vi "CLD 1_Elapsed_Time_Express_ZLK_Solution.vi"(6 "Stop VI":bool, 8 "error in":errorcluster, 9 "Auto Reset":bool=TRUE, 10 "Reset Button":bool, 11 "Time Target (s)":dbl=2.0) -> (0 "error out":errorcluster, 2 "Time has Elapsed":bool, 3 "Elapsed Time":string="0  00:00:00")   [LabVIEW 2023]
doc: "LabVIEW CLD 1 Exercise"
uses:
  b5ba48de-fc09-4468-998c-c920f8fd6674.vi
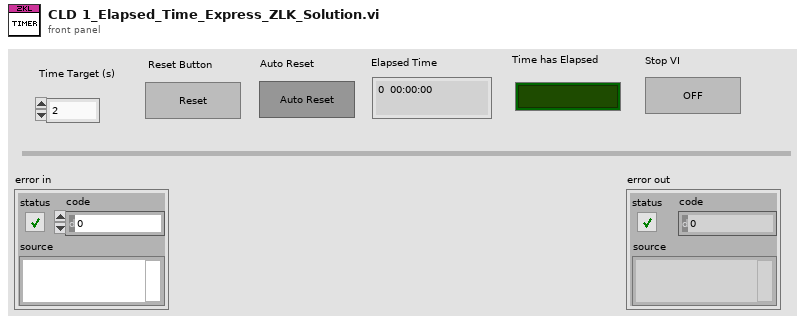
[diagram p1: front panel]
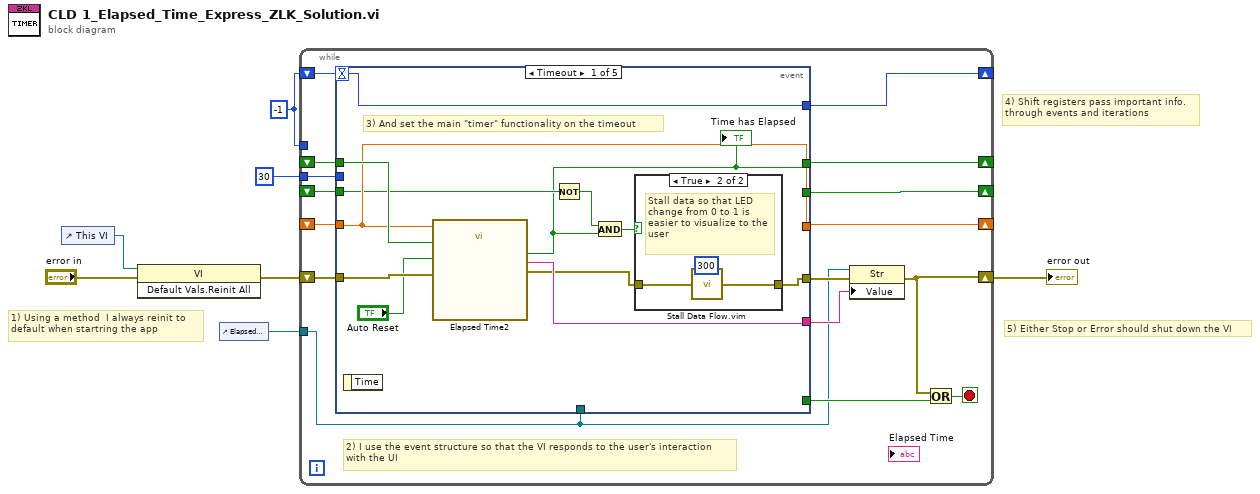
[diagram p0: block diagram]
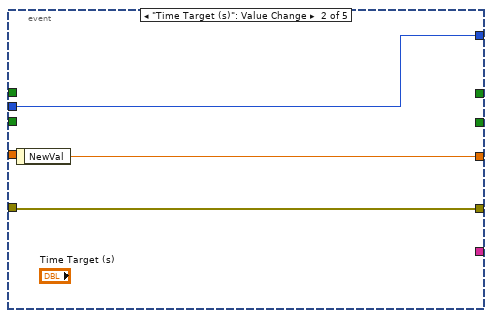
[diagram p3: hidden frame]
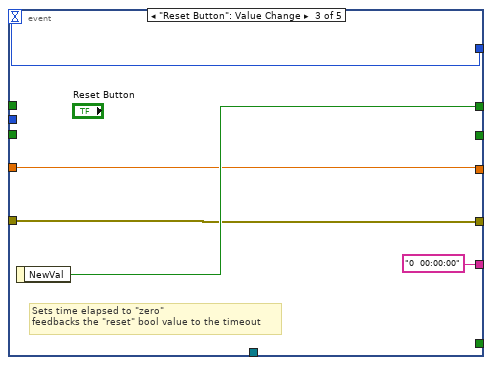
[diagram p4: hidden frame]
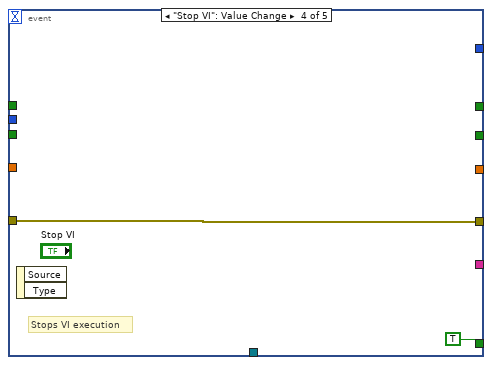
[diagram p5: hidden frame]
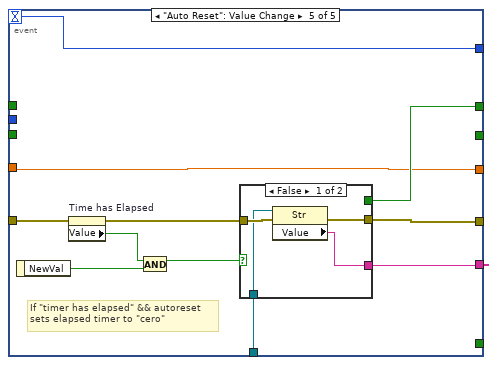
[diagram p6: hidden frame]
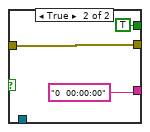
[diagram p7: hidden frame]
diagram:
  w2 = -1
  # "5) Either Stop or Error should shut down the VI"
  # "4) Shift registers pass important info.\nthrough events and iterations"
  # "1) Using a method  I always reinit to \ndefault when startring the app"
  n1 = control-ref of="This VI"() -> (w4:refnum<vi>)
  n2 = invoke class="VI" method="Default Vals.Reinit All"(reference=w4, error in="error in") -> (error out=w5:errorcluster)  [unwired: 1 in, 2 out]
  n3 = control-ref of="Elapsed Time"() -> (w3:refnum<vi>)
  n4 = while {
    shift-right: [w15] -> w6
    shift-left: w5 -> [w23]
    shift-right: [w22] -> _
    shift-left: _ -> [w21]
    shift-right: [w13] -> _
    shift-left: w2 -> [w20]
    shift-right: [w18] -> _
    shift-left: _ -> [w17]
    tunnel: w3 -> [w8]
    tunnel: w2 -> [_]
    tunnel: 30 -> [w12]
    shift-right: [w10] -> _
    shift-left: _ -> [w9]
    stop <- w19 stop-if-true
    # "2) I use the event structure so that the VI responds to the user's interaction\nwith the UI"
    n5 = event shown="[0] Timeout" {
      selector: _ -> [_ _ _ _ _]
      dyn-events: _ -> [_ _ _ _ _]
      timeout: w20 -> [w30 _ w47 _ w53]
      tunnel: w23 -> [w35 w41 w44 w48 w60]
      tunnel: [w32 w42 w45 _ w52] -> w22
      tunnel: w21 -> [w32 _ w45 _ w52]
      tunnel: [w30 w40 w47 _ w53] -> w13
      tunnel: [_ _ w46 _ w54] -> w18
      tunnel: w17 -> [w33 _ _ _ _]
      tunnel: [w31 _ "0  00:00:00" ("Elapsed Time") _ w51] -> w16
      tunnel: [w29 w41 w44 w48 w57] -> w14
      tunnel: w12 -> [_ w40 _ _ _]
      tunnel: [_ _ _ TRUE ("Stop VI") _] -> w11
      tunnel: [w25 _ _ _ _] -> w10
      tunnel: w9 -> [w26 _ _ _ _]
      tunnel: w8 -> [_ _ _ _ w50]
      event Timeout {
        # "3) And set the main \"timer\" functionality on the timeout"
        n6 = event-data() -> ()  [unwired: 1 in, 1 out]
        n7 = call "Elapsed Time2"("Time Target (s)"=w32, "Reset"=w33, "Auto Reset"="Auto Reset", "error in (no error)"=w35) -> ("Time has Elapsed"=w25:bool, "Elapsed Time Text"=w31:string, "error out"=w28:errorcluster)  [unwired: 8 in, 5 out]
        "Time has Elapsed" <- w25
        n8 = Not(x=w26) -> (.not. x?=w24:bool)
        n9 = And(x=w24, y=w25) -> (x .and. y?=w27:bool)
        n10 = case shown="True" w27 {
          tunnel: [w36 w38] -> w29
          tunnel: w28 -> [w36 w39]
          frame False {
          }
          frame True {
            # "Stall data so that LED\nchange from 0 to 1 is\neasier to visualize to the\nuser"
            n11 = call "Stall Data Flow.vim"("value in"=w39, "milliseconds to wait"=300) -> ("value out"=w38:errorcluster)  [unwired: 1 out]
          }
        }
      }
      event "Time Target (s)": Value Change {
        n12 = event-data() -> ("NewVal"=w42:dbl)  [unwired: 1 in]
      }
      event "Reset Button": Value Change {
        # "Sets time elapsed to \"zero\"\nfeedbacks the \"reset\" bool value to the timeout"
        n13 = event-data() -> ("NewVal"=w46:bool)  [unwired: 1 in]
      }
      event "Stop VI": Value Change {
        # "Stops VI execution"
        n14 = event-data() -> ()  [unwired: 1 in, 2 out]
      }
      event "Auto Reset": Value Change {
        # "If \"timer has elapsed\" && autoreset\nsets elapsed timer to \"cero\""
        n15 = event-data() -> ("NewVal"=w59:bool)  [unwired: 1 in]
        n16 = property on="Time has Elapsed" class="Bool (strict)"(error in=w60) -> (error out=w58:errorcluster, "Value"=w55:bool)  [unwired: 1 in, 1 out]
        n17 = And(x=w55, y=w59) -> (x .and. y?=w56:bool)
        n18 = case shown="False" w56 {
          tunnel: w58 -> [w64 w67]
          tunnel: [w63 w67] -> w57
          tunnel: [_ TRUE ("NewVal")] -> w54
          tunnel: [w61 "0  00:00:00" ("Elapsed Time")] -> w51
          tunnel: w50 -> [w62 _]
          frame False {
            n19 = property class="Str"(reference=w62, error in=w64) -> (error out=w63:errorcluster, "Value"=w61:string)  [unwired: 1 out]
          }
          frame True {
          }
        }
      }
    }
    n20 = property class="Str"(reference=w8, error in=w14, "Value"=w16) -> (error out=w15:errorcluster)  [unwired: 1 out]
    n21 = Or(x=w15, y=w11) -> (x .or. y?=w19:bool)
  }
  "error out" <- w6
